vi "Close Driver.vi"(8 "error in (no error)":errorcluster) -> (0 "error out":errorcluster)   [LabVIEW 2015, in "TPVG_DLL.lvlib"]
doc: "Use to close the link between the DLL interface and the\nKernel mode driver\n\nWORD CLASS_DECLSPEC CloseDriver( void );\n\n------------------------------------------------------------------\nWritten by: Dang Lam"
uses:
  TPVG_DLL.lvlib
  TPVG_DLL.dll
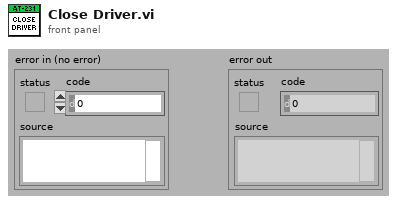
[diagram p1: front panel]
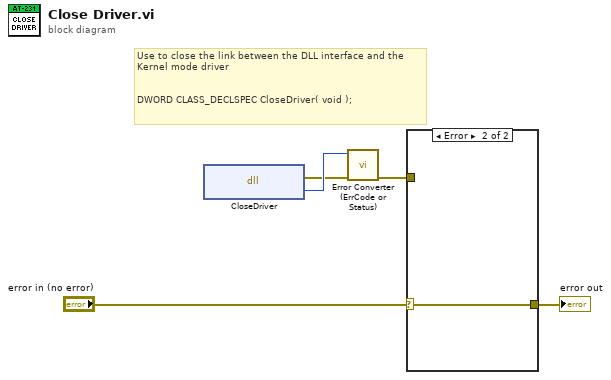
[diagram p0: block diagram]
diagram:
  # "Use to close the link between the DLL interface and the\nKernel mode driver\n\n\nDWORD CLASS_DECLSPEC CloseDriver( void );"
  n1 = dll-call lib="\\\\Mac\\Home/Desktop/imt_test_app 28-06-2012/TPVG_DLL.dll" fn="CloseDriver"() -> (error out=w4:errorcluster, "Return"=w5:u32)  [unwired: 3 in, 1 out]
  n2 = call "Error Converter (ErrCode or Status).vi"("error in (no error)"=w4, "error code"=w5) -> ("error out"=w1:errorcluster)  [unwired: 9 in]
  n3 = case shown="Error" "error in (no error)" {
    selector: "error in (no error)" -> [_ w7]
    tunnel: [w6 w7] -> w2
    tunnel: w1 -> [w6 _]
    frame No Error {
    }
    frame Error {
    }
  }
  "error out" <- w2
